vi "First Derivate.vi"(8 "deltaX":dbl format="%.2f", 9 "differentiator":dbl[](array[numeric]) format="%.2f", 11 "Y[n]":dbl[](array[numeric]) format="%.2f") -> (3 "dY/dX[n]":dbl[](array[numeric]) format="%.2f")   [LabVIEW 2017, in "SoundVib_TachProcess.lvlib"]
uses:
  <vilib>/addons/Sound and Vibration/Order Analysis/Tach Process/SoundVib_TachProcess.lvlib
  <vilib>/Analysis/2dsp.llb/1D Convolution (DBL).vi
  <vilib>/Analysis/NI_AALPro.lvlib
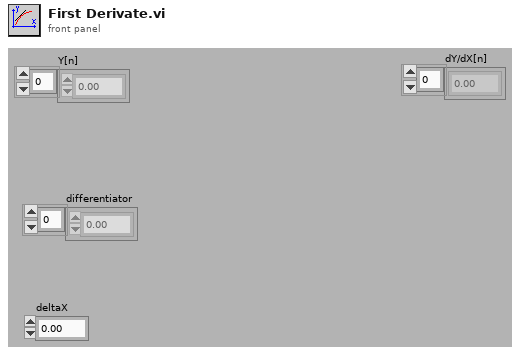
[diagram p1: front panel]
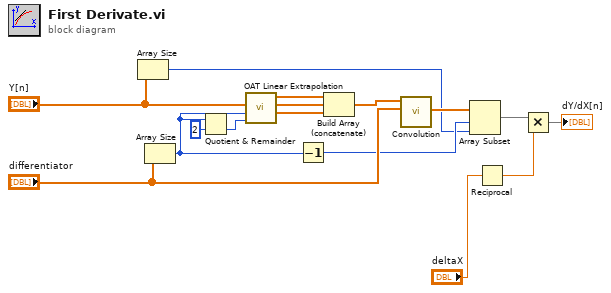
[diagram p0: block diagram]
diagram:
  n1 = Array Size(array="Y[n]") -> (size(s)=w1:i32)
  n2 = Array Size(array="differentiator") -> (size(s)=w14:i32)
  n3 = Quotient & Remainder(x=w14, y=2) -> (floor(x/y)=w3:i32)  [unwired: 1 out]
  n4 = call <vilib>:"OAT Linear Extrapolation.vi"("extrapolation length"=w3, "modal length"=w14, "X[n]"="Y[n]") -> ("final"=w5:dbl[], "X[n] out"=w6:dbl[], "initail"=w4:dbl[])  [unwired: 6 in]
  n5 = Decrement(x=w14) -> (x-1=w9:i32)
  n6 = Build Array (concatenate)(w4, w6, w5) -> (w11:dbl[])
  n7 = call-poly <vilib>:"Convolution.vi"("Y"="differentiator", "X"=w11) -> ("X * Y"=w12:dbl[])  [unwired: 8 in, 1 out]
  n8 = Array Subset(array=w12, index=w9, length=w1) -> (w13:dbl[])
  n9 = Reciprocal(x="deltaX") -> (1/x=w8:dbl)
  n10 = Multiply(x=w13, y=w8) -> (x*y=→"dY/dX[n]":dbl[])
